vi "readIniFile.vi"(8 "Error In":errorcluster, 11 "File Path Control":path) -> (0 "Error Out":errorcluster, 3 "Value":string[][](array[string]))   [LabVIEW 2018]
uses:
  controls/iniDriverSelectorEnum.ctl
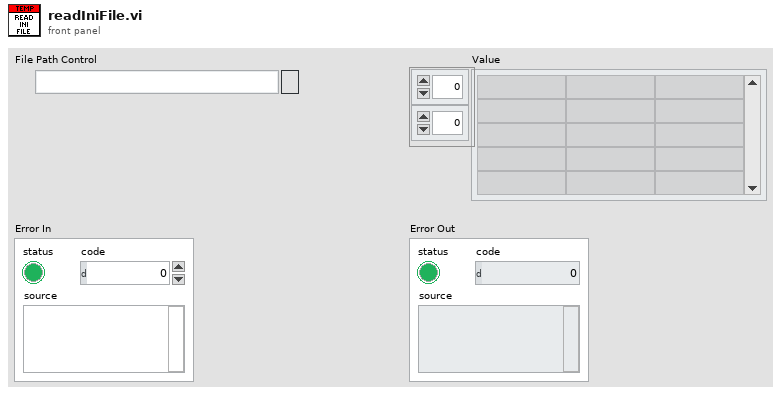
[diagram p1: front panel]
types:
  T1 = typedef "iniDriverSelectorEnum.ctl" = enum16{"open", "Write", "Read", "close"}
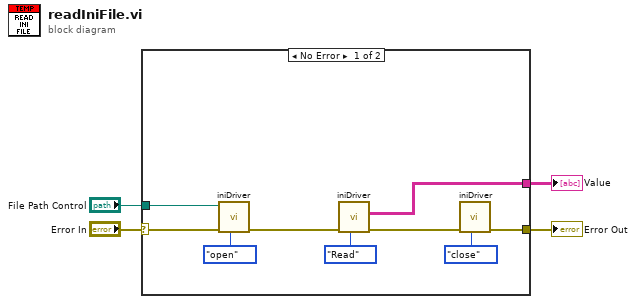
[diagram p0: block diagram]
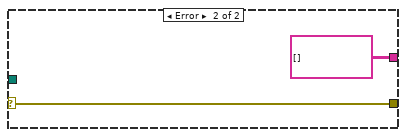
[diagram p2: hidden frame]
diagram:
  n1 = case shown="No Error" "Error In" {
    selector: "Error In" -> [w8 w15]
    tunnel: [w7 w15] -> w3
    tunnel: "File Path Control" -> [w6 _]
    tunnel: [w5 string[][] [] ("Value Out")] -> w1
    frame No Error {
      n2 = call "iniDriver.vi"("INI Options"=iniDriverSelectorEnum."open", "Error In"=w8, "File Path In"=w6) -> ("Error Out"=w10:errorcluster)  [unwired: 6 in, 2 out]
      n3 = call "iniDriver.vi"("INI Options"=iniDriverSelectorEnum."Read", "Error In"=w10) -> ("Error Out"=w9:errorcluster, "Value Out"=w5:string[][])  [unwired: 7 in, 1 out]
      n4 = call "iniDriver.vi"("INI Options"=iniDriverSelectorEnum."close", "Error In"=w9) -> ("Error Out"=w7:errorcluster)  [unwired: 7 in, 2 out]
    }
    frame Error {
    }
  }
  "Error Out" <- w3
  "Value" <- w1
